vi "Untitled 1.vi"(7 "VISA resource name":refnum<visa-resource-name>) -> (6 "Speed":dbl)   [LabVIEW 2016]
uses:
  <vilib>/Instr/_visa.llb/VISA Configure Serial Port (Instr).vi
panel:
  out "x-y":u32
  out "error out 2":errorcluster
  out "read buffer":string
  out "error out":errorcluster
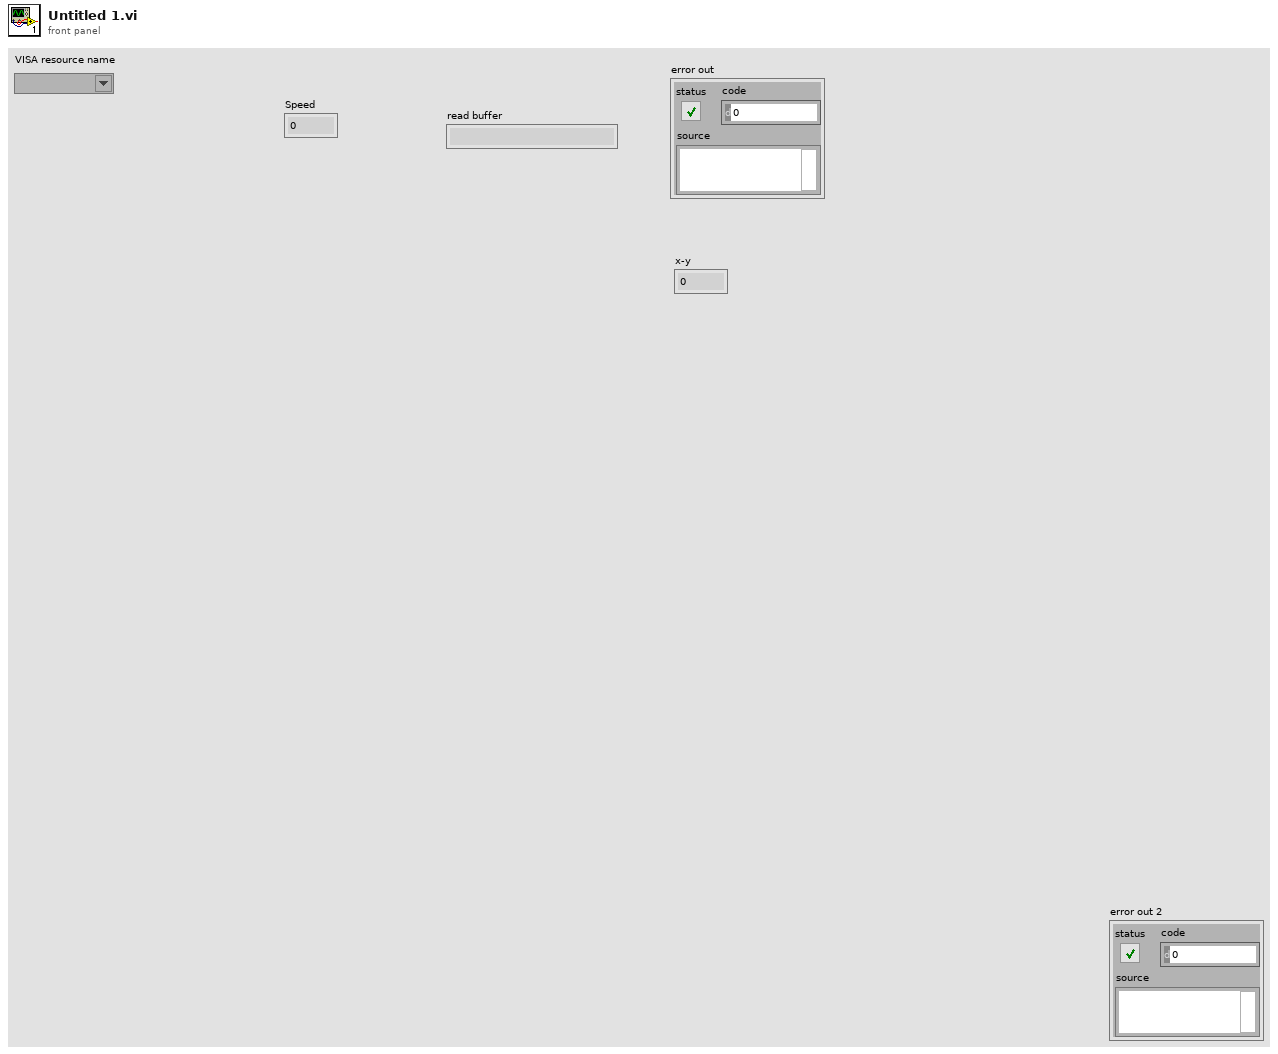
[diagram p1: front panel]
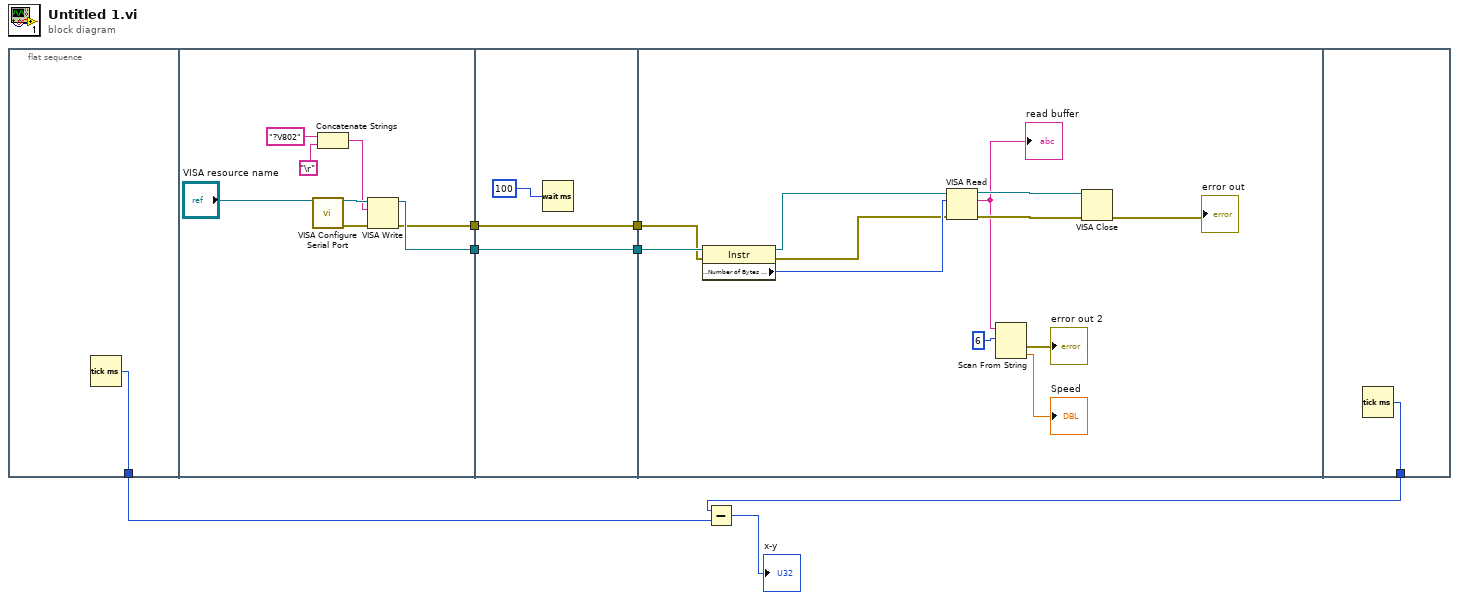
[diagram p0: block diagram]
diagram:
  n1 = flat-sequence {
    tunnel: [w8] -> w6
    tunnel: [w10] -> w3
    tunnel: [w9] -> w2
    tunnel: [w18] -> w4
    tunnel: w3 -> [w18]
    tunnel: w2 -> [w17]
    tunnel: [w17] -> w1
    tunnel: w4 -> [w24]
    tunnel: w1 -> [w20]
    tunnel: [w32] -> w7
    frame #0 {
      n2 = Tick Count (ms)() -> (millisecond timer value=w8:u32)
    }
    frame #1 {
      n3 = call-poly "VISA Configure Serial Port"("VISA resource name"="VISA resource name") -> ("VISA resource name out"=w14:refnum<visa-resource-name>, "error out"=w15:errorcluster)  [unwired: 13 in]
      n4 = Concatenate Strings("?V802" ("write buffer"), "\r") -> (w13:string)
      n5 = VISA Write(VISA resource name=w14, write buffer=w13, error in (no error)=w15) -> (VISA resource name out=w10:refnum<visa-resource-name>, error out=w9:errorcluster)  [unwired: 1 out]
    }
    frame #2 {
      n6 = Wait (ms)(milliseconds to wait=u32 100) -> ()  [unwired: 1 out]
    }
    frame #3 {
      n7 = property class="Instr"(reference=w24, error in=w20) -> (reference out=w22:refnum<visa-resource-name>, error out=w21:errorcluster, "Serial Settings:Number of Bytes at Serial Port"=w23:u32)
      n8 = VISA Read(VISA resource name=w22, byte count=w23, error in (no error)=w21) -> (VISA resource name out=w30:refnum<visa-resource-name>, read buffer=w25:string, error out=w31:errorcluster)  [unwired: 1 out]
      "read buffer" <- w25
      n9 = Scan From String(input string=w25, initial scan location=u32 6) -> (error out=→"error out 2":errorcluster, output 1=→"Speed":dbl)  [unwired: 3 in, 2 out]
      n10 = VISA Close(VISA resource name=w30, error in (no error)=w31) -> (error out=→"error out":errorcluster)
    }
    frame #4 {
      n11 = Tick Count (ms)() -> (millisecond timer value=w32:u32)
    }
  }
  n12 = Subtract(x=w7, y=w6) -> (x-y=→"x-y":u32)
